vi "ep_Manage Aggregation Interval.vi"(0 "aggregation settings":T1={"interval"=1, "interval unit"=enum."Runs", "synchronization of intervals"=enum."Not synchronized", "algorithm"=enum."Average"}, 1 "restart (F)":bool, 5 "data time stamp":timestamp, 11 "error in (no error)":errorcluster) -> (4 "aggregated data time stamp":timestamp, 6 "aggregated data valid?":bool, 8 "restart aggregation?":bool, 10 "runs":u32, 15 "error out":errorcluster)   [LabVIEW 2011, in "NI_EP_Power Quality.lvlib"]
uses:
  <vilib>/addons/Electrical Power/PQ/NI_EP_Power Quality.lvlib
  <vilib>/addons/Electrical Power/PQ/Common/Controls/ep_Aggregation Settings.ctl
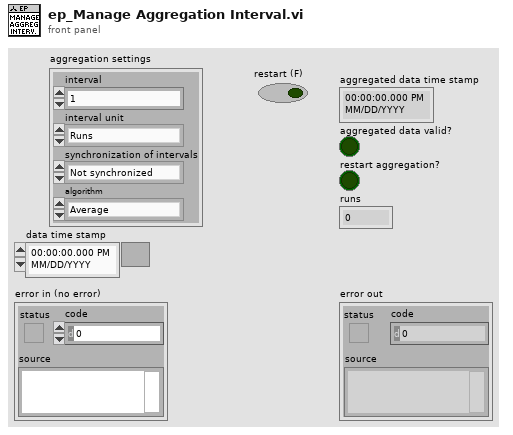
[diagram p1: front panel]
types:
  T1 = typedef "NI_EP_Power Quality.lvlib/ep_Aggregation Settings.ctl" = cluster{"interval":u32, "interval unit":enum16{"Runs", "Seconds", "Minutes", "Hours", "Days", "Weeks"}, "synchronization of intervals":enum16{"Not synchronized", "Interval rounded"}, "algorithm":enum16{"Average", "RMS"}}
  T2 = enum16{"Runs", "Seconds", "Minutes", "Hours", "Days", "Weeks"}
  T3 = typedef "LVDateTimeRec.ctl" = cluster{"fractional second":dbl, "second":i32, "minute":i32, "hour":i32, "day of month":i32, "month":i32, "year":i32, "day of week":i32, "day of year":i32, "DST":i32}
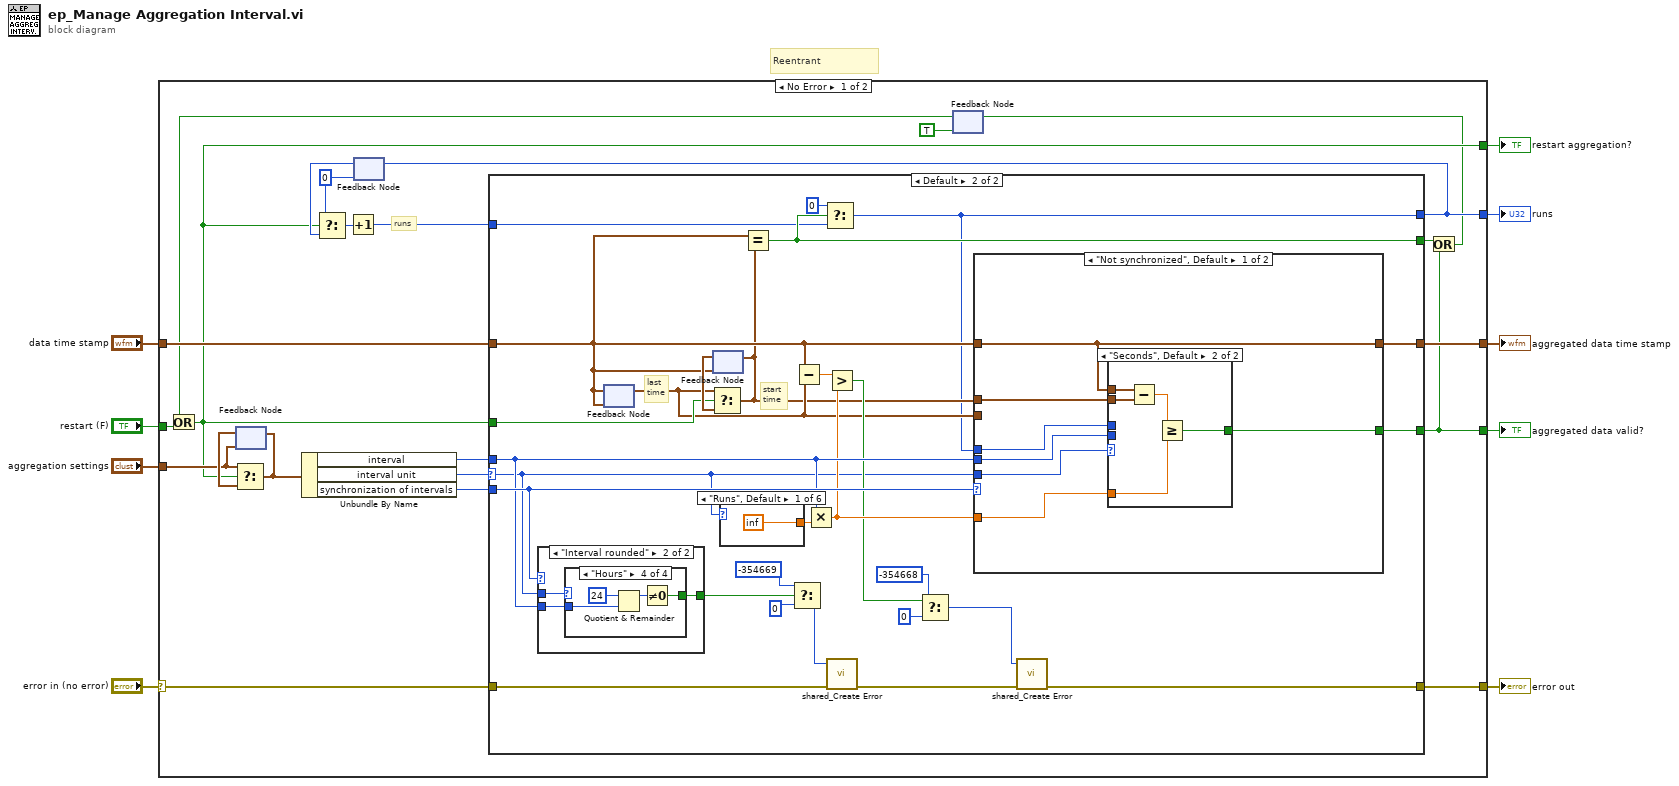
[diagram p0: block diagram]
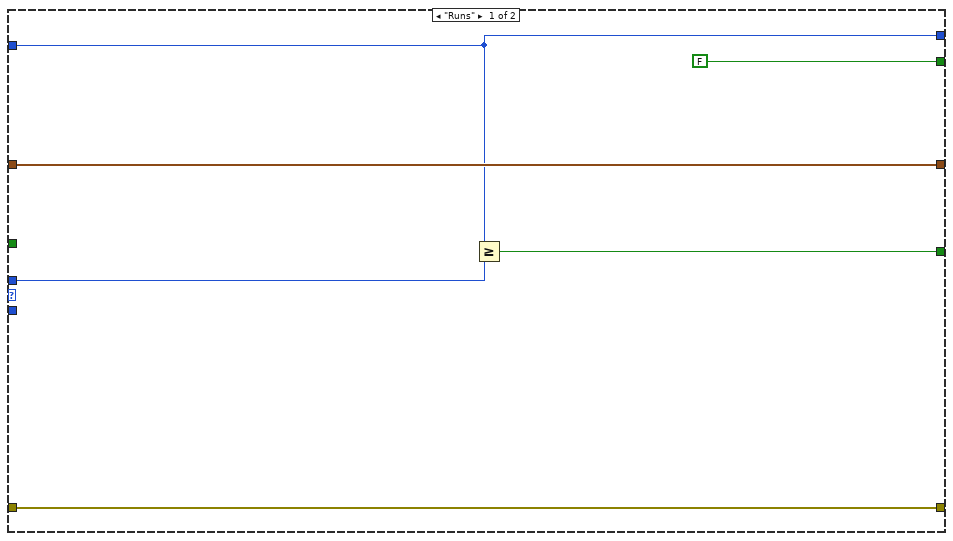
[diagram p2: hidden frame]
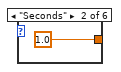
[diagram p3: hidden frame]
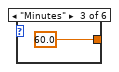
[diagram p4: hidden frame]
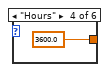
[diagram p5: hidden frame]
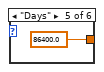
[diagram p6: hidden frame]
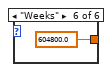
[diagram p7: hidden frame]
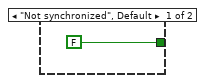
[diagram p8: hidden frame]
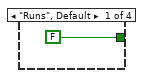
[diagram p9: hidden frame]
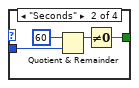
[diagram p10: hidden frame]
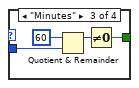
[diagram p11: hidden frame]
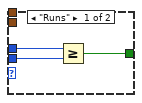
[diagram p12: hidden frame]
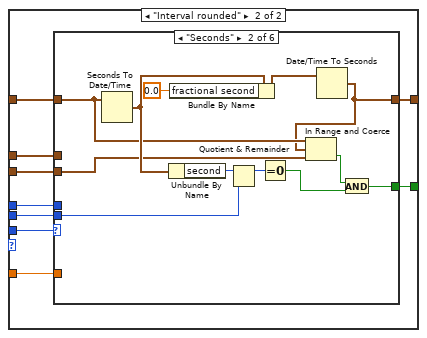
[diagram p13: hidden frame]
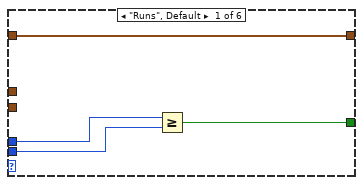
[diagram p14: hidden frame]
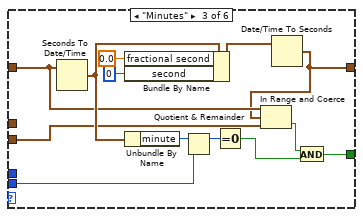
[diagram p15: hidden frame]
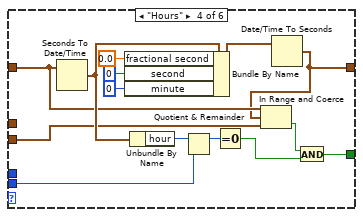
[diagram p16: hidden frame]
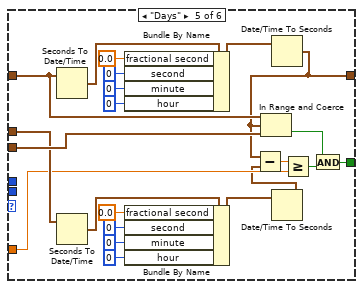
[diagram p17: hidden frame]
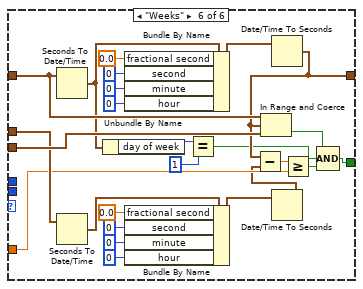
[diagram p18: hidden frame]
diagram:
  # "Reentrant"
  n1 = case shown="No Error" "error in (no error)" {
    selector: "error in (no error)" -> [w26 w203]
    tunnel: [w16 _] -> w9
    tunnel: [w10 _] -> w8
    tunnel: [w31 _] -> w7
    tunnel: "restart (F)" -> [w23 _]
    tunnel: "aggregation settings" -> [w22 _]
    tunnel: "data time stamp" -> [w29 _]
    tunnel: [w27 w203] -> w3
    tunnel: [w13 _] -> w1
    frame No Error {
      w15 = u32 0
      # "runs"
      n2 = feedback #1(w22) -> (w24:T1)
      n3 = feedback #2(w15) -> (w14:u32)
      n4 = feedback #3(TRUE) -> (w20:bool)
      n5 = Or(x=w20, y=w23) -> (x .or. y?=w13:bool)
      n6 = Select(t=w22, s=w13, f=w24) -> (s? t:f=w21:T1)
      n7 = feedback-in #1(w21) -> ()
      n8 = Unbundle By Name(w21) -> ("interval"=w28:u32, "interval unit"=w19:T2, "synchronization of intervals"=w30:enum16{"Not synchronized", "Interval rounded"})
      n9 = Select(t=w15, s=w13, f=w14) -> (s? t:f=w18:u32)
      n10 = Increment(x=w18) -> (x+1=w17:u32)
      n11 = case shown="Default" w19 {
        selector: w19 -> [_ w54]
        tunnel: [w37 w65] -> w31
        tunnel: w30 -> [_ w63]
        tunnel: w29 -> [w37 w52]
        tunnel: w28 -> [w32 w60]
        tunnel: [w34 w39] -> w27
        tunnel: w26 -> [w34 w43]
        tunnel: w13 -> [_ w57]
        tunnel: [w36 w56] -> w10
        tunnel: w17 -> [w33 w48]
        tunnel: [FALSE w49] -> w12
        tunnel: [w33 w47] -> w16
        frame "Runs" {
          n12 = Greater Or Equal?(x=w33, y=w32) -> (x >= y?=w36:bool)
        }
        frame Default {
          # "start\ntime"
          # "last\ntime"
          n13 = case shown="\"Interval rounded\"" w63 {
            tunnel: w54 -> [_ w75]
            tunnel: w60 -> [_ w74]
            tunnel: [FALSE w73] -> w62
            frame "Not synchronized", Default {
            }
            frame "Interval rounded" {
              n14 = case shown="\"Hours\"" w75 {
                tunnel: w74 -> [_ w79 w83 w87]
                tunnel: [FALSE w77 w81 w85] -> w73
                frame "Runs", Default {
                }
                frame "Seconds" {
                  n15 = Quotient & Remainder(x=u32 60, y=w79) -> (x-y*floor(x/y)=w78:u32)  [unwired: 1 out]
                  n16 = Not Equal To 0?(x=w78) -> (x != 0?=w77:bool)
                }
                frame "Minutes" {
                  n17 = Quotient & Remainder(x=u32 60, y=w83) -> (x-y*floor(x/y)=w82:u32)  [unwired: 1 out]
                  n18 = Not Equal To 0?(x=w82) -> (x != 0?=w81:bool)
                }
                frame "Hours" {
                  n19 = Quotient & Remainder(x=u32 24, y=w87) -> (x-y*floor(x/y)=w86:u32)  [unwired: 1 out]
                  n20 = Not Equal To 0?(x=w86) -> (x != 0?=w85:bool)
                }
              }
            }
          }
          n21 = feedback-in #4(w52) -> ()
          n22 = feedback #4(w52) -> (w53:timestamp)
          n23 = feedback #5(w52) -> (w64:timestamp)
          n24 = Select(t=w53, s=w57, f=w64) -> (s? t:f=w51:timestamp)
          n25 = feedback-in #5(w51) -> ()
          n26 = case shown="\"Runs\", Default" w54 {
            tunnel: [inf 1.0 60.0 3600.0 86400.0 604800.0] -> w59
            frame "Runs", Default {
            }
            frame "Seconds" {
            }
            frame "Minutes" {
            }
            frame "Hours" {
            }
            frame "Days" {
            }
            frame "Weeks" {
            }
          }
          n27 = Equal?(x=w52, y=w51) -> (x = y?=w49:bool)
          n28 = Select(t=-354669, s=w62, f=0 ("error code (0)")) -> (s? t:f=w44:i32)
          n29 = Subtract(x=w52, y=w53) -> (x-y=w61:dbl)
          n30 = Multiply(x=w60, y=w59) -> (x*y=w58:dbl)
          n31 = Select(t=u32 0, s=w49, f=w48) -> (s? t:f=w47:u32)
          n32 = Greater?(x=w61, y=w58) -> (0:w55:bool)
          n33 = call <vilib>:"shared_Create Error.vi"("error in (no error)"=w43, "error code (0)"=w44) -> ("error out"=w40:errorcluster)  [unwired: 9 in]
          n34 = Select(t=-354668, s=w55, f=0 ("error code (0)")) -> (s? t:f=w38:i32)
          n35 = case shown="\"Not synchronized\", Default" w63 {
            tunnel: w54 -> [w95 w112]
            tunnel: w60 -> [w94 w111]
            tunnel: w47 -> [w93 w110]
            tunnel: [w92 w109] -> w56
            tunnel: w52 -> [w91 w108]
            tunnel: [w91 w107] -> w65
            tunnel: w51 -> [w90 w106]
            tunnel: w53 -> [_ w105]
            tunnel: w58 -> [w89 w104]
            frame "Not synchronized", Default {
              n36 = case shown="\"Seconds\", Default" w95 {
                tunnel: w93 -> [w98 _]
                tunnel: w94 -> [w97 _]
                tunnel: [w96 w101] -> w92
                tunnel: w90 -> [_ w103]
                tunnel: w91 -> [_ w102]
                tunnel: w89 -> [_ w99]
                frame "Runs" {
                  n37 = Greater Or Equal?(x=w98, y=w97) -> (x >= y?=w96:bool)
                }
                frame "Seconds", Default {
                  n38 = Subtract(x=w102, y=w103) -> (x-y=w100:dbl)
                  n39 = Greater Or Equal?(x=w100, y=w99) -> (x >= y?=w101:bool)
                }
              }
            }
            frame "Interval rounded" {
              n40 = case shown="\"Seconds\"" w112 {
                tunnel: w110 -> [w116 _ _ _ _ _]
                tunnel: w111 -> [w115 w126 w139 w153 _ _]
                tunnel: [w114 w120 w133 w147 w172 w198] -> w109
                tunnel: w108 -> [w113 w121 w134 w148 w173 w199]
                tunnel: [w113 w117 w130 w144 w159 w185] -> w107
                tunnel: w106 -> [_ _ _ _ w162 w188]
                tunnel: w105 -> [_ w122 w135 w149 w174 w200]
                tunnel: w104 -> [_ _ _ _ w160 w186]
                frame "Runs", Default {
                  n41 = Greater Or Equal?(x=w116, y=w115) -> (x >= y?=w114:bool)
                }
                frame "Seconds" {
                  n42 = Seconds To Date/Time(time stamp (now)=w121) -> (date time rec=w123:T3)  [unwired: 1 in]
                  n43 = Unbundle By Name(w123) -> ("second"=w128:i32)
                  n44 = Bundle By Name(cluster=w123, "fractional second"=0.0) -> (w124:T3)
                  n45 = Quotient & Remainder(x=w128, y=w126) -> (x-y*floor(x/y)=w127:u32)  [unwired: 1 out]
                  n46 = Equal To 0?(x=w127) -> (x = 0?=w119:bool)
                  n47 = Date/Time To Seconds(2:w124) -> (0:w117:timestamp)  [unwired: 1 in]
                  n48 = In Range and Coerce(upper limit=w121, x=w117, lower limit=w122) -> (In Range?=w118:bool)  [unwired: 1 out]
                  n49 = And(x=w118, y=w119) -> (x .and. y?=w120:bool)
                }
                frame "Minutes" {
                  n50 = Seconds To Date/Time(time stamp (now)=w134) -> (date time rec=w136:T3)  [unwired: 1 in]
                  n51 = Bundle By Name(cluster=w136, "fractional second"=0.0, "second"=0) -> (w137:T3)
                  n52 = Unbundle By Name(w136) -> ("minute"=w141:i32)
                  n53 = Quotient & Remainder(x=w141, y=w139) -> (x-y*floor(x/y)=w140:u32)  [unwired: 1 out]
                  n54 = Equal To 0?(x=w140) -> (x = 0?=w132:bool)
                  n55 = Date/Time To Seconds(2:w137) -> (0:w130:timestamp)  [unwired: 1 in]
                  n56 = In Range and Coerce(upper limit=w134, x=w130, lower limit=w135) -> (In Range?=w131:bool)  [unwired: 1 out]
                  n57 = And(x=w131, y=w132) -> (x .and. y?=w133:bool)
                }
                frame "Hours" {
                  n58 = Seconds To Date/Time(time stamp (now)=w148) -> (date time rec=w150:T3)  [unwired: 1 in]
                  n59 = Bundle By Name(cluster=w150, "fractional second"=0.0, "second"=0, "minute"=0) -> (w151:T3)
                  n60 = Unbundle By Name(w150) -> ("hour"=w155:i32)
                  n61 = Quotient & Remainder(x=w155, y=w153) -> (x-y*floor(x/y)=w154:u32)  [unwired: 1 out]
                  n62 = Equal To 0?(x=w154) -> (x = 0?=w146:bool)
                  n63 = Date/Time To Seconds(2:w151) -> (0:w144:timestamp)  [unwired: 1 in]
                  n64 = In Range and Coerce(upper limit=w148, x=w144, lower limit=w149) -> (In Range?=w145:bool)  [unwired: 1 out]
                  n65 = And(x=w145, y=w146) -> (x .and. y?=w147:bool)
                }
                frame "Days" {
                  n66 = Seconds To Date/Time(time stamp (now)=w173) -> (date time rec=w175:T3)  [unwired: 1 in]
                  n67 = Seconds To Date/Time(time stamp (now)=w162) -> (date time rec=w165:T3)  [unwired: 1 in]
                  n68 = Bundle By Name(cluster=w175, "fractional second"=0.0, "second"=0, "minute"=0, "hour"=0) -> (w176:T3)
                  n69 = Bundle By Name(cluster=w165, "fractional second"=0.0, "second"=0, "minute"=0, "hour"=0) -> (w164:T3)
                  n70 = Date/Time To Seconds(2:w176) -> (0:w159:timestamp)  [unwired: 1 in]
                  n71 = In Range and Coerce(upper limit=w173, x=w159, lower limit=w174) -> (In Range?=w157:bool)  [unwired: 1 out]
                  n72 = Date/Time To Seconds(2:w164) -> (0:w158:timestamp)  [unwired: 1 in]
                  n73 = Subtract(x=w159, y=w158) -> (x-y=w161:dbl)
                  n74 = Greater Or Equal?(x=w161, y=w160) -> (x >= y?=w156:bool)
                  n75 = And(x=w157, y=w156) -> (x .and. y?=w172:bool)
                }
                frame "Weeks" {
                  n76 = Seconds To Date/Time(time stamp (now)=w199) -> (date time rec=w182:T3)  [unwired: 1 in]
                  n77 = Seconds To Date/Time(time stamp (now)=w188) -> (date time rec=w191:T3)  [unwired: 1 in]
                  n78 = Unbundle By Name(w182) -> ("day of week"=w181:i32)
                  n79 = Bundle By Name(cluster=w182, "fractional second"=0.0, "second"=0, "minute"=0, "hour"=0) -> (w201:T3)
                  n80 = Bundle By Name(cluster=w191, "fractional second"=0.0, "second"=0, "minute"=0, "hour"=0) -> (w190:T3)
                  n81 = Equal?(x=w181, y=1 ("x")) -> (x = y?=w179:bool)
                  n82 = Date/Time To Seconds(2:w201) -> (0:w185:timestamp)  [unwired: 1 in]
                  n83 = In Range and Coerce(upper limit=w199, x=w185, lower limit=w200) -> (In Range?=w180:bool)  [unwired: 1 out]
                  n84 = Date/Time To Seconds(2:w190) -> (0:w184:timestamp)  [unwired: 1 in]
                  n85 = Subtract(x=w185, y=w184) -> (x-y=w187:dbl)
                  n86 = Greater Or Equal?(x=w187, y=w186) -> (x >= y?=w183:bool)
                  n87 = Compound Arithmetic op=AND(w180, w179, w183) -> (w198:bool)
                }
              }
            }
          }
          n88 = call <vilib>:"shared_Create Error.vi"("error in (no error)"=w40, "error code (0)"=w38) -> ("error out"=w39:errorcluster)  [unwired: 9 in]
        }
      }
      n89 = feedback-in #2(w16) -> ()
      n90 = Or(x=w12, y=w10) -> (x .or. y?=w11:bool)
      n91 = feedback-in #3(w11) -> ()
    }
    frame Error {
    }
  }
  "aggregated data valid?" <- w8
  "aggregated data time stamp" <- w7
  "runs" <- w9
  "error out" <- w3
  "restart aggregation?" <- w1
